vi "Init Dll.vi"(10 "en_hard_watchdog":u32, 11 "en_log":u32) -> (3 "function return":i32)   [LabVIEW 2021, in "vmmso.lvlib"]
doc: "DLL_API int WINAPI InitDll(unsigned int en_log, unsigned int en_hard_watchdog);"
uses:
  vmmso.lvlib
  vmmso.dll
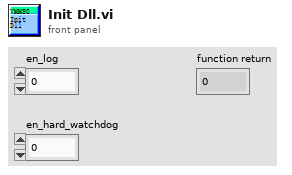
[diagram p1: front panel]
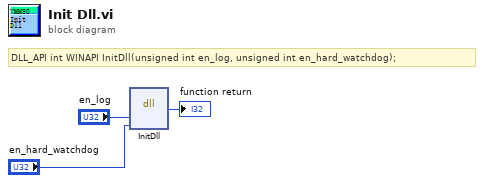
[diagram p0: block diagram]
diagram:
  # "DLL_API int WINAPI InitDll(unsigned int en_log, unsigned int en_hard_watchdog);"
  n1 = dll-call lib="D:/labviewdemo/LabviewDemo 21/vmmso/vmmso.*" fn="InitDll"("en_log"="en_log", "en_hard_watchdog"="en_hard_watchdog") -> (→"function return":i32)  [unwired: 5 in, 2 out]
